vi "Script Find current Error Codes.vi"(8 "error in":errorcluster, 11 "Library in":refnum<vi>) -> (0 "error out":errorcluster, 1 "All Error VIS":path[](array[path]), 2 "Error and Descriptions Table":string[][](array[string]), 3 "Library out":refnum<vi>)   [LabVIEW 2020, in "ConstantErrorsMaker.lvlib"]
uses:
  ConstantErrorsMaker.lvlib
  <vilib>/Utility/traverseref.llb/TRef TravTarget.ctl
  <vilib>/Utility/traverseref.llb/VI Scripting - Traverse.lvlib
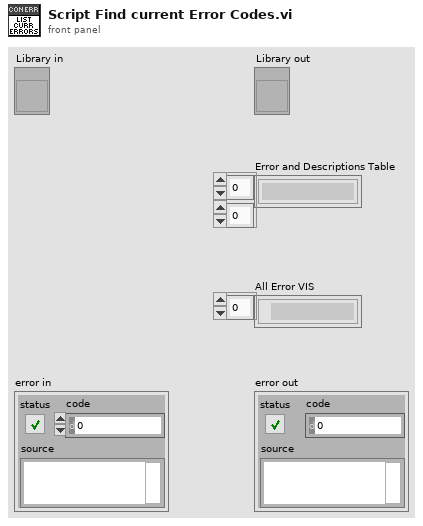
[diagram p1: front panel]
types:
  T1 = typedef "TRef TravTarget.ctl" = enum16{"FP", "BD", "Other"}
  T2 = cluster{"Clipped Error Description":string, "Full Error Description":string, "code":i32, "Family":string, "Custom Description":string, "Is Error":bool, "Types":variant[], "Include Call Chain?":bool, "Error Text Visible":bool}
  T3 = cluster{"Library Version":cluster{"Major":u16, "Minor":u16, "Fix":u16, "Build":u16}, "State":variant}
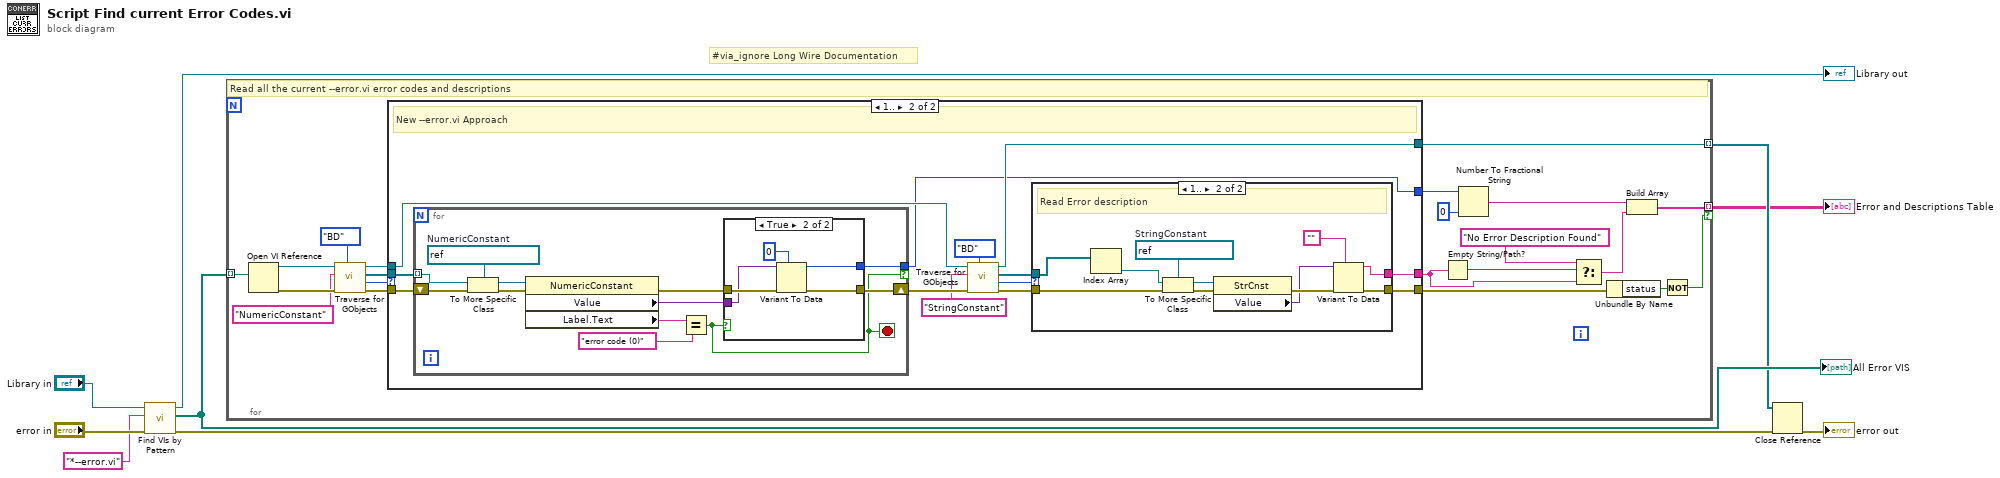
[diagram p0: block diagram]
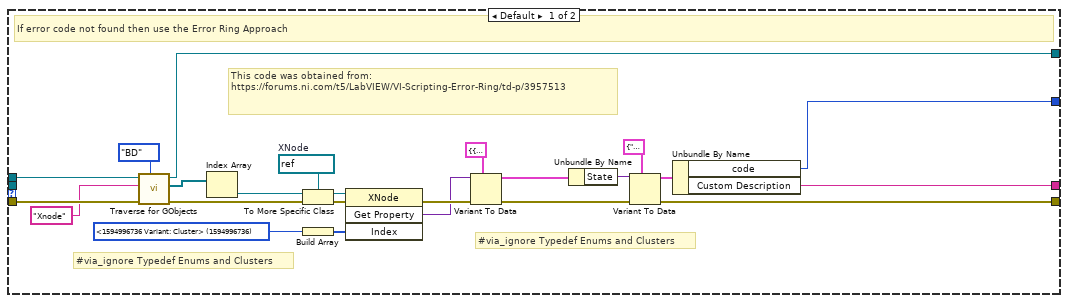
[diagram p2: hidden frame]
diagram:
  # "#via_ignore Long Wire Documentation"
  n1 = call "Find VIs by Pattern.vi"("error in"="error in", "pattern"="*--error.vi", "Library in"="Library in") -> ("error out"=w8:errorcluster, "All Files in Dir"=w4:path[], "Library out"=→"Library out":refnum<vi>)  [unwired: 6 in]
  "All Error VIS" <- w4
  n2 = for {
    tunnel: w4 -> [w21] mode=indexing
    tunnel: [w20] -> w3 mode=indexing
    tunnel: [w15] -> w1 mode=indexing if=w14
    # "Read all the current --error.vi error codes and descriptions"
    n3 = Open VI Reference(vi path=w21) -> (vi reference=w25:refnum<vi>, error out=w29:errorcluster)  [unwired: 5 in]
    n4 = call <vilib>:"Traverse for GObjects.vi"("Traverse Target"=TRef_TravTarget."BD", "error in (no error)"=w29, "Class Name"="NumericConstant", "VI Refnum"=w25) -> ("error out"=w30:errorcluster, "# of Refs"=w23:i32, "References"=w26:refnum<vi>[], "dup VI Refnum"=w22:refnum<vi>)  [unwired: 4 in]
    n5 = case shown="1.." w23 {
      tunnel: [w33 w55] -> w17
      tunnel: [w51 w66] -> w28
      tunnel: w30 -> [w54 w65]
      tunnel: w26 -> [_ w63]
      tunnel: w22 -> [w46 w58]
      tunnel: [w32 w57] -> w12
      tunnel: [w31 w56] -> w20
      frame Default {
        w42 = u32 1594996736 items=["<1594996736 Variant: Cluster>"=1594996736, "<1594996767 Diagram RefNum>"=1594996737, "<1594996738 ProjectItem Refnum>"=1594996738, "<1594996739 Boolean>"=1594996739, "<1594996740 Boolean>"=1594996740, "<1594996741 Boolean>"=1594996741, "<1594996742 String: .html file name>"=1594996742, "<1594996743 Help Path>"=1594996743, "<1594996744 String: Tip Strip>"=1594996744, "<1594996745 Boolean>"=1594996745, "<104204298 Boolean>"=104204298, "AutoSize To Fit Contents?"=104204288, "Basic Object Flags"=103983116, "Bounds"=103983107, "Bounds:Area Height"=103983109, "Bounds:Area Width"=103983108, "Breakpoint Status"=104173580, "Clump Num"=104173572, "Content Rect"=104204293, "Description"=104173570, "Diagrams[]"=104204291, "Fire Count"=104173574, "Fix Contents"=104204297, "Frame Size"=104204290, "Icon"=104173576, "Is Asynchronous"=104173575, "Is Break Point Set"=104173571, "Is Run At Any Loop"=104173578, "Is Wizard Locked"=103983117, "Label"=104173569, "Master Bounds Rect"=103983115, "Position"=103983104, "Position:Left"=103983105, "Position:Top"=103983106, "Resize Info:Can Resize Horizontally"=103983119, "Resize Info:Can Resize Vertically"=103983120, "Resize Info:Include In Resize"=103983122, "Resize Info:Name in Resize Dialog"=103983121, "Selected"=103983113, "Shared Clones:Automatic Allocation Strategy Enabled"=104204295, "Shared Clones:Pre-Allocate"=104204296, "Short Count"=104173573, "Style"=104173577, "Target Syntax Checking"=104204292, "Terminals[]"=104173568, "Total Bounds Rect"=103983114, "Tunnels[]"=104204289, "UID"=103983123]
        w45 = refnum<vi> refnum  # XNode
        # "#via_ignore Typedef Enums and Clusters"
        # "#via_ignore Typedef Enums and Clusters"
        # "This code was obtained from:\nhttps://forums.ni.com/t5/LabVIEW/VI-Scripting-Error-Ring/td-p/3957513"
        # "If error code not found then use the Error Ring Approach"
        n6 = call <vilib>:"Traverse for GObjects.vi"("Traverse Target"=TRef_TravTarget."BD", "error in (no error)"=w54, "Class Name"="Xnode", "VI Refnum"=w46) -> ("error out"=w53:errorcluster, "References"=w44:refnum<vi>[], "dup VI Refnum"=w31:refnum<vi>)  [unwired: 4 in, 1 out]
        n7 = Index Array(array=w44) -> (element=w43:refnum<vi>)  [unwired: 1 in]
        n8 = To More Specific Class(target class=w45, reference=w43, error in=w53) -> (specific class reference=w41:refnum<vi>, error out=w52:errorcluster)
        n9 = Build Array(w42) -> (w40:u32[])
        n10 = invoke class="XNode" method="Get Property"(reference=w41, error in=w52, "Index"=w40) -> (error out=w50:errorcluster, "GetProperty"=w35:variant)  [unwired: 1 in, 2 out]
        n11 = Variant To Data(error in=w50, type=T3 {"Library Version"={"Major"=0, "Minor"=0, "Fix"=0, "Build"=0}, "State"=variant} ("output cluster"), Variant=w35) -> (data=w39:T3, error out=w49:errorcluster)
        n12 = Unbundle By Name(w39) -> ("State"=w37:variant)
        n13 = Variant To Data(error in=w49, type=T2 {"Clipped Error Description"="", "Full Error Description"="", "code"=0, "Family"="", "Custom Description"="", "Is Error"=TRUE, "Types"=[], "Include Call Chain?"=TRUE, "Error Text Visible"=TRUE} ("State"), Variant=w37) -> (data=w34:T2, error out=w51:errorcluster)
        n14 = Unbundle By Name(w34) -> ("code"=w33:i32, "Custom Description"=w32:string)
      }
      frame 1.. {
        # "New --error.vi Approach"
        n15 = for {
          tunnel: w63 -> [w75] mode=indexing
          tunnel: [w69] -> w55 if=w68
          shift-right: [w76] -> w64
          shift-left: w65 -> [w79]
          stop <- w68 stop-if-true
          w74 = refnum<vi> refnum  # NumericConstant
          n16 = To More Specific Class(target class=w74, reference=w75, error in=w79) -> (specific class reference=w73:refnum<vi>, error out=w78:errorcluster)
          n17 = property class="NumericConstant"(reference=w73, error in=w78) -> (error out=w77:errorcluster, "Value"=w70:variant, "Label.Text"=w72:string)  [unwired: 1 out]
          n18 = Equal?(x=w72, y="error code (0)") -> (x = y?=w68:bool)
          n19 = case shown="True" w68 {
            tunnel: w70 -> [_ w82]
            tunnel: w77 -> [w80 w85]
            tunnel: [w80 w84] -> w76
            tunnel: [_ w81] -> w69
            frame False {
            }
            frame True {
              n20 = Variant To Data(error in=w85, type=0, Variant=w82) -> (data=w81:i32, error out=w84:errorcluster)
            }
          }
        }
        n21 = call <vilib>:"Traverse for GObjects.vi"("Traverse Target"=TRef_TravTarget."BD", "error in (no error)"=w64, "Class Name"="StringConstant", "VI Refnum"=w58) -> ("error out"=w67:errorcluster, "# of Refs"=w59:i32, "References"=w62:refnum<vi>[], "dup VI Refnum"=w56:refnum<vi>)  [unwired: 4 in]
        n22 = case shown="1.." w59 {
          tunnel: [_ w93] -> w57
          tunnel: [w86 w97] -> w66
          tunnel: w67 -> [w86 w96]
          tunnel: w62 -> [_ w88]
          frame Default {
          }
          frame 1.. {
            w92 = refnum<vi> refnum  # StringConstant
            # "Read Error description"
            n23 = Index Array(array=w88) -> (element=w87:refnum<vi>)  [unwired: 1 in]
            n24 = To More Specific Class(target class=w92, reference=w87, error in=w96) -> (specific class reference=w91:refnum<vi>, error out=w95:errorcluster)
            n25 = property class="StrCnst"(reference=w91, error in=w95) -> (error out=w94:errorcluster, "Value"=w90:variant)  [unwired: 1 out]
            n26 = Variant To Data(error in=w94, type="", Variant=w90) -> (data=w93:string, error out=w97:errorcluster)
          }
        }
      }
    }
    n27 = Empty String/Path?(string/path=w12) -> (empty?=w13:bool)
    n28 = Number To Fractional String(number=w17, precision (6)=i16 0) -> (F-format string=w18:string)  [unwired: 2 in]
    n29 = Select(t="No Error Description Found", s=w13, f=w12) -> (s? t:f=w11:string)
    n30 = Unbundle By Name(w28) -> ("status"=w19:bool)
    n31 = Build Array(w18, w11) -> (w15:string[])
    n32 = Not(x=w19) -> (.not. x?=w14:bool)
  }
  "Error and Descriptions Table" <- w1
  n33 = Close Reference(reference=w3, error in (no error)=w8) -> (error out=→"error out":errorcluster)
